vi "Normalize Angle.vi"(8 "Initial Angle":dbl, 11 "Angle in r":dbl) -> (3 "Angle out r":dbl)   [LabVIEW 2019]
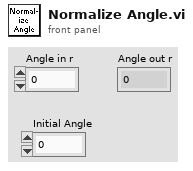
[diagram p1: front panel]
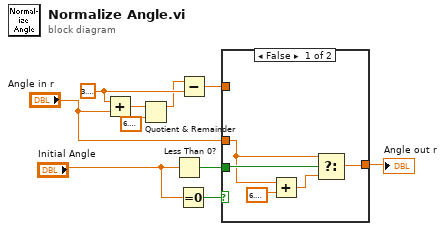
[diagram p0: block diagram]
diagram:
  w10 = 3.141592653589793
  n1 = Add(x=w10, y="Angle in r") -> (x+y=w7:dbl)
  n2 = Quotient & Remainder(x=w7, y=6.283185307179586) -> (x-y*floor(x/y)=w8:dbl)  [unwired: 1 out]
  n3 = Less Than 0?(x="Initial Angle") -> (x < 0?=w6:bool)
  n4 = Equal To 0?(x="Initial Angle") -> (x = 0?=w1:bool)
  n5 = Subtract(x=w8, y=w10) -> (x-y=w4:dbl)
  n6 = case shown="False" w1 {
    tunnel: w6 -> [w15 _]
    tunnel: [w13 w16] -> w5
    tunnel: w4 -> [_ w16]
    tunnel: "Angle in r" -> [w12 _]
    frame False {
      n7 = Add(x=w12, y=6.283185307179586) -> (x+y=w11:dbl)
      n8 = Select(t=w12, s=w15, f=w11) -> (s? t:f=w13:dbl)
    }
    frame True {
    }
  }
  "Angle out r" <- w5
